vi "GetCRC8.vi"(8 "错误输入（无错误）":errorcluster, 11 "xData":u8[](array[numeric]) format="0x%x") -> (0 "错误输出":errorcluster, 3 "CRC8":u8 format="0x%x")   [LabVIEW 2020]
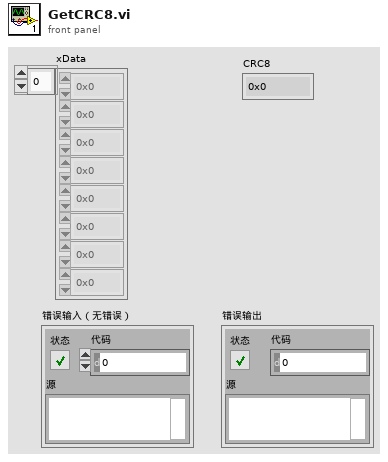
[diagram p1: front panel]
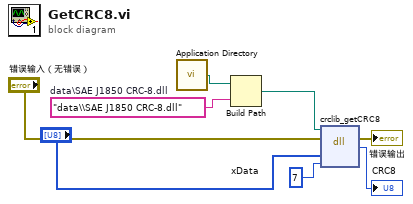
[diagram p0: block diagram]
diagram:
  w3 = "data\\SAE J1850 CRC-8.dll"  # data\SAE J1850 CRC-8.dll
  n1 = call <vilib>:"Application Directory.vi"() -> ("Application Directory"=w4:path)
  n2 = Build Path(base path=w4, name or relative path=w3) -> (appended path=w2:path)
  n3 = dll-call lib="PTH2aabs CUsersFeng项目HengLongtrunk性能试验台SourcesdllSAE J1850 CRC-8.dll" fn="crclib_getCRC8"(path in=w2, error in="错误输入（无错误）", "xData"="xData", "xDataLen"=u16 7) -> (error out=→"错误输出":errorcluster, "返回类型"=→"CRC8":u8)  [unwired: 3 in, 1 out]
